vi "Read ExpTime SV.vi"(8 "error in (no error)":errorcluster, 11 "Integrator in":refnum<class "Integrator.lvclass">) -> (0 "error out":errorcluster, 2 "ExpTime SV":refnum<k21>, 3 "Integrator out":refnum<class "Integrator.lvclass">)   [LabVIEW 2016, in "Integrator.lvclass"]
uses:
  Integrator.lvclass
  Integrator.lvclass/Integrator.ctl
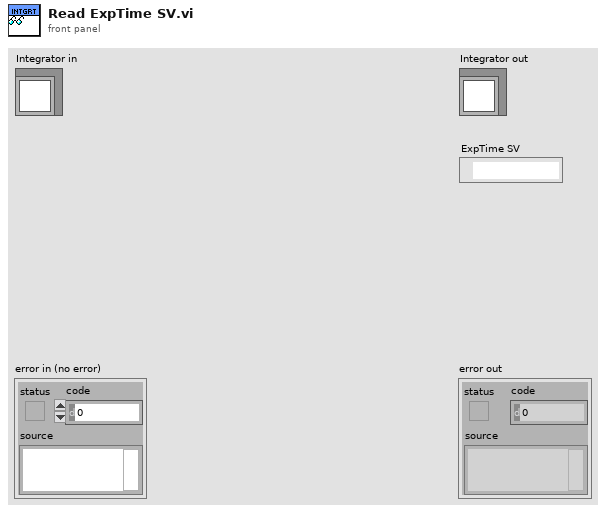
[diagram p1: front panel]
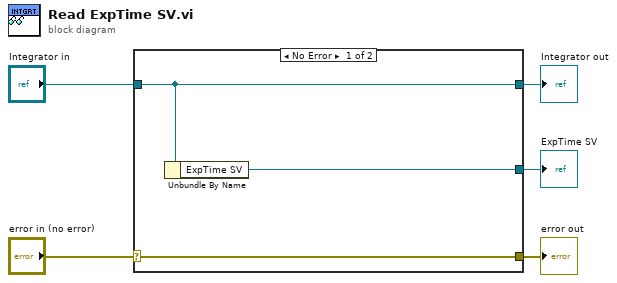
[diagram p0: block diagram]
diagram:
  n1 = case shown="No Error" "error in (no error)" {
    selector: "error in (no error)" -> [w8 w9]
    tunnel: [w8 w9] -> w4
    tunnel: [w7 w10] -> w2
    tunnel: "Integrator in" -> [w7 w10]
    tunnel: [w6 _] -> w1
    frame No Error {
      n2 = Unbundle By Name(w7) -> ("ExpTime SV"=w6:refnum<k21>)
    }
    frame Error {
    }
  }
  "error out" <- w4
  "Integrator out" <- w2
  "ExpTime SV" <- w1
